vi "DigSeqLogic_Off_Delay.vi"(8 "Time":dbl=-1.0, 9 "Delay":dbl=1.0, 11 "Input":bool) -> (1 "Remain":dbl, 3 "Output":bool)   [LabVIEW 2019, in "Trajectory_Library.lvlib"]
doc: "This VI implements a digital \"off delay\". The output becomes TRUE when the input goes TRUE. The output remains TRUE for a specified time after the input goes FALSE.\n\nInputs:\n - Input -- Boolean input value\n - Delay -- Off delay time in seconds.\n - Time -- Continously counting system time, Seconds. If not wired the FPGA time will be used.\n\nOutputs:\n - Output -- Boolean output value with the off delay applied\n - Remain -- Time remaining for this value to be on, seconds. Value will be 0 to Delay input value."
uses:
  Trajectory_Library.lvlib
  <vilib>/Utility/semaphor.llb/Obtain Semaphore Reference.vi
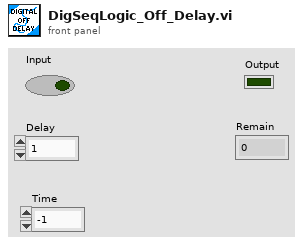
[diagram p1: front panel]
types:
  T1 = typedef "Trajectory_Library.lvlib/TIMER.ctl" = cluster{"StartTime":dbl, "Accumulated TIme":dbl, "Running":bool, "semaphore":T2}
  T2 = typedef "Semaphore RefNum" = refnum<k1>
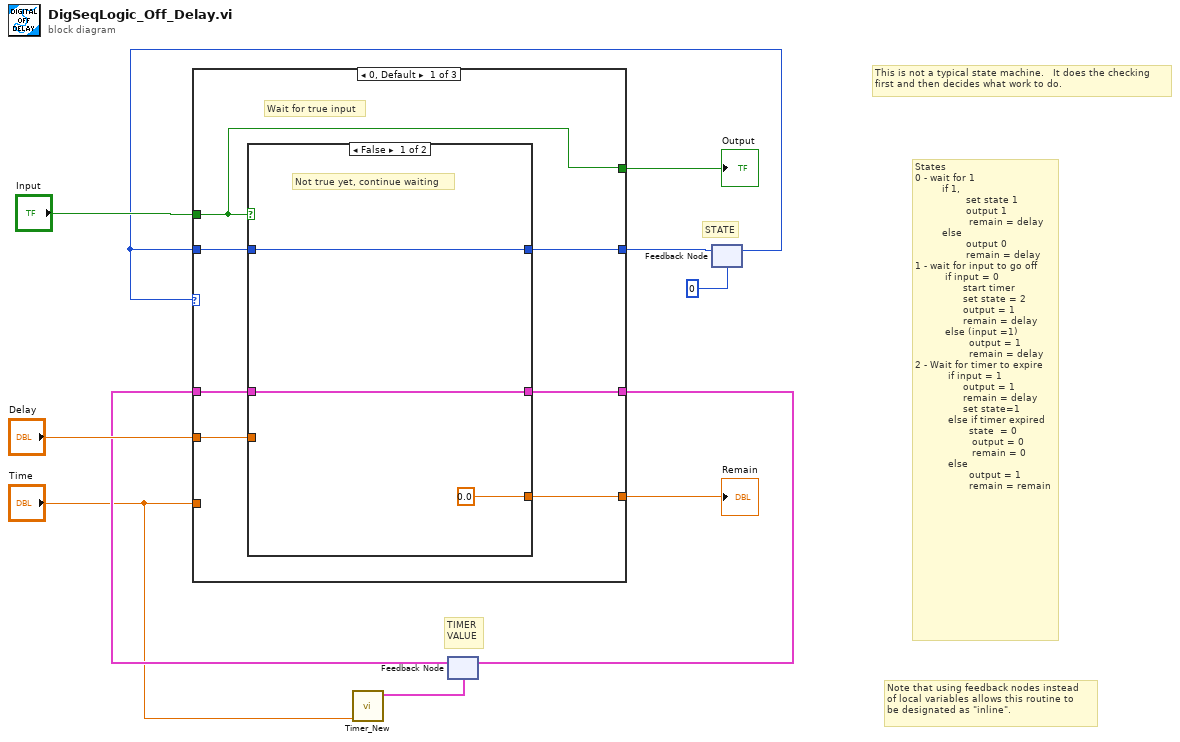
[diagram p0: block diagram]
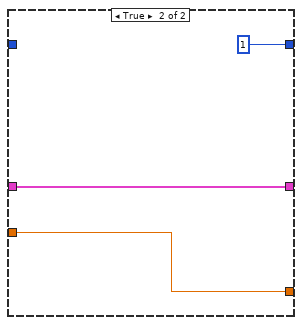
[diagram p2: hidden frame]
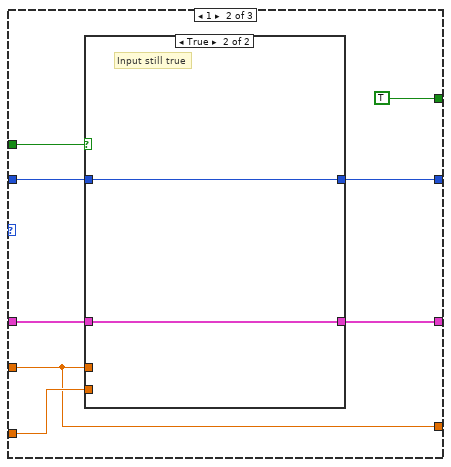
[diagram p3: hidden frame]
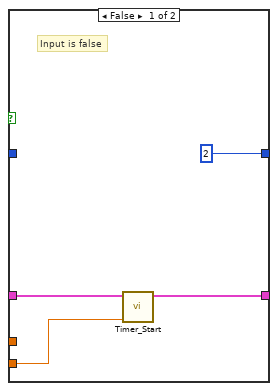
[diagram p4: hidden frame]
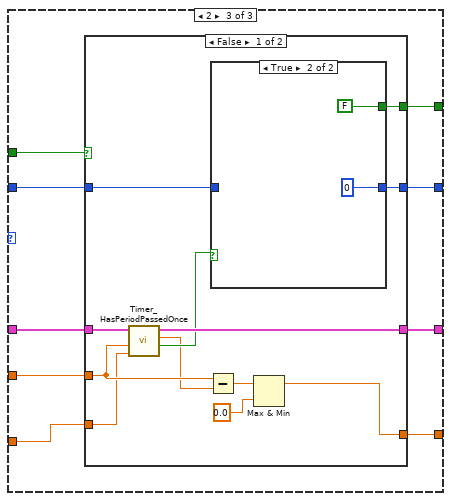
[diagram p5: hidden frame]
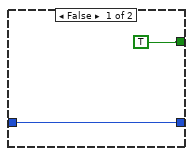
[diagram p6: hidden frame]
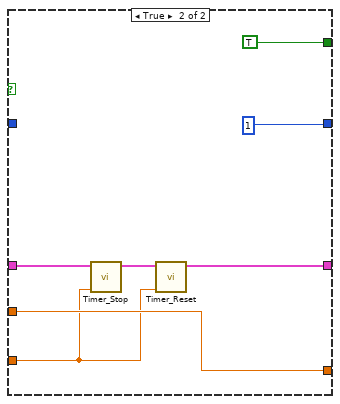
[diagram p7: hidden frame]
diagram:
  # "This is not a typical state machine.   It does the checking\nfirst and then decides what work to do."
  # "TIMER\nVALUE"
  # "Note that using feedback nodes instead\nof local variables allows this routine to\nbe designated as \"inline\"."
  # "STATE"
  # "States \n0 - wait for 1\n         if 1, \n                 set state 1\n                 output 1\n                  remain = delay\n         else\n                 output 0\n                 remain = delay    \n1 - wait for input to go off\n          if input = 0\n                start timer\n                set state = 2\n                output = 1\n                remain = delay\n          else (input =1)\n                  output = 1\n                  remain = delay\n2 - Wait for timer to expire\n           if input = 1\n                output = 1\n                remain = delay\n                set state=1\n           else if timer expired\n                  state  = 0\n                   output = 0\n                   remain = 0\n           else \n                  output = 1\n                  remain = remain"
  n1 = call "Timer_New.vi"("Pass_Through_Time"="Time") -> ("TIMER"=w2:T1)  [unwired: 10 in]
  n2 = feedback #1(w2) -> (w4:T1)
  n3 = feedback #2(0 ("State")) -> (w6:i32)
  n4 = case shown="0, Default" w6 {
    tunnel: "Delay" -> [w16 w30 w45]
    tunnel: "Time" -> [_ w31 w42]
    tunnel: [w18 TRUE w46] -> w10
    tunnel: [w17 w30 w44] -> w9
    tunnel: w4 -> [w13 w25 w43]
    tunnel: "Input" -> [w18 w32 w47]
    tunnel: [w15 w28 w41] -> w7
    tunnel: w6 -> [w14 w27 w40]
    tunnel: [w12 w26 w39] -> w3
    frame 0, Default {
      # "Wait for true input"
      n5 = case shown="False" w18 {
        tunnel: [0.0 ("Delay") w24] -> w17
        tunnel: w16 -> [_ w24]
        tunnel: [w20 1 ("State")] -> w15
        tunnel: w14 -> [w20 _]
        tunnel: w13 -> [w19 w22]
        tunnel: [w19 w22] -> w12
        frame False {
          # "Not true yet, continue waiting"
        }
        frame True {
        }
      }
    }
    frame 1 {
      n6 = case shown="True" w32 {
        tunnel: w30 -> [_ _]
        tunnel: w31 -> [w33 _]
        tunnel: [2 ("State") w38] -> w28
        tunnel: w27 -> [_ w38]
        tunnel: [w34 w37] -> w26
        tunnel: w25 -> [w35 w37]
        frame False {
          # "Input is false"
          n7 = call "Timer_Start.vi"("Pass_Through_Time"=w33, "in Timer"=w35) -> ("out Timer"=w34:T1)  [unwired: 9 in]
        }
        frame True {
          # "Input still true"
        }
      }
    }
    frame 2 {
      n8 = case shown="False" w47 {
        tunnel: [w59 TRUE] -> w46
        tunnel: w45 -> [w51 w69]
        tunnel: [w53 w69] -> w44
        tunnel: w43 -> [w56 w67]
        tunnel: w42 -> [w48 w64]
        tunnel: [w58 1 ("State")] -> w41
        tunnel: w40 -> [w57 _]
        tunnel: [w55 w65] -> w39
        frame False {
          n9 = call "Timer_HasPeriodPassedOnce.vi"("Pass_Through_Time"=w48, "Period"=w51, "in Timer"=w56) -> ("Expired"=w54:bool, "CurrentTImer"=w50:dbl, "out Timer"=w55:T1)  [unwired: 6 in]
          n10 = Subtract(x=w51, y=w50) -> (x-y=w49:dbl)
          n11 = case shown="True" w54 {
            tunnel: [TRUE FALSE] -> w59
            tunnel: [w60 0 ("State")] -> w58
            tunnel: w57 -> [w60 _]
            frame False {
            }
            frame True {
            }
          }
          n12 = Max & Min(x=w49, y=0.0) -> (max(x,y)=w53:dbl)  [unwired: 1 out]
        }
        frame True {
          n13 = call "Timer_Stop.vi"("Pass_Through_Time"=w64, "in Timer"=w67) -> ("out Timer"=w66:T1)  [unwired: 9 in]
          n14 = call "Timer_Reset.vi"("Pass_Through_Time"=w64, "in TIMER"=w66) -> ("out TIMER"=w65:T1)  [unwired: 9 in]
        }
      }
    }
  }
  "Remain" <- w9
  "Output" <- w10
  n15 = feedback-in #1(w3) -> ()
  n16 = feedback-in #2(w7) -> ()
